vi "ScopeRead.vi"(6 "CalArray":u8[](array[numeric]), 7 "BufferSize":i32=2048, 8 "error in (no error)":errorcluster caption="错误输入（无错误）", 9 "Range":dbl=5.0, 10 "ch":i32, 11 "handle":u64) -> (0 "error out":errorcluster caption="错误输出", 1 "voltages":dbl[](array[numeric]), 2 "function return":i32, 3 "handle out":u64, 5 "backsize out":i32)   [LabVIEW 2018]
doc: "Read Scope data"
uses:
  InstrumentsPlayground.lvlib
panel:
  out "CalArray out":u8[](array[numeric])
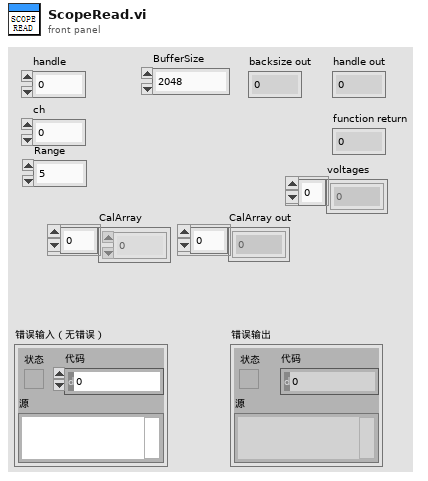
[diagram p1: front panel]
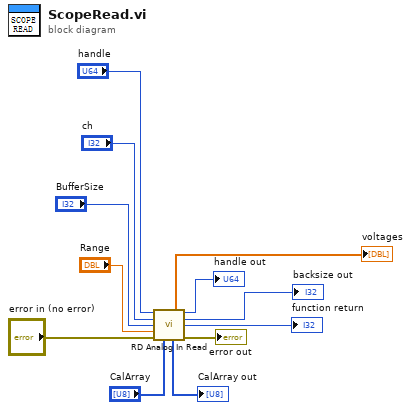
[diagram p0: block diagram]
diagram:
  n1 = call "RD Analog In Read.vi"("handle"="handle", "ch"="ch", "size"="BufferSize", "range"="Range", "error in (no error)"="error in (no error)", "CalArray"="CalArray") -> ("RxBuffer out"=→"voltages":dbl[], "handle out"=→"handle out":u64, "backsize out"=→"backsize out":i32, "function return"=→"function return":i32, "CalArray out"=→"CalArray out":u8[], "error out"=→"error out":errorcluster)  [unwired: 4 in]
